vi "afonin_et7026(1) — 18.09.2023.vi"() -> ()   [LabVIEW 2012]
panel:
  out "error out":errorcluster
  out "Торр":dbl format="%#_2g"
  out "Па":dbl format="%#_2e"
  out "мбар":dbl format="%#_2g"
  out "Торр":dbl(graph)
  out "Waveform Chart":dbl(graph)
  in  "Remote Port":u16=502
  in  "Remote IP for 7026":string="127.0.0.1"
  in  "Stop":bool
  out "AI":u16[](array[numeric])
  out "DI":bool[](array[boolean]) caption="Slave Discrete Inputs"
  in  "DO":bool[](array[boolean])=[FALSE, FALSE, FALSE, FALSE] caption="Coils to Write"
  in  "AO":u16[](array[numeric])=[0, 0, 0, 0] caption="Registers to Write"
  # "192.168.0.122"
  # "Data to write to the slave"
  # "Slave Read-only Registers"
  # "DO 0"
  # "DO 1"
  # "DI 0"
  # "DI 1"
  # "AO 0"
  # "AO 1"
  # "AI 0"
  # "AI 1"
  # "AI 2"
  # "AI 3"
  # "AI 4"
  # "AI 5"
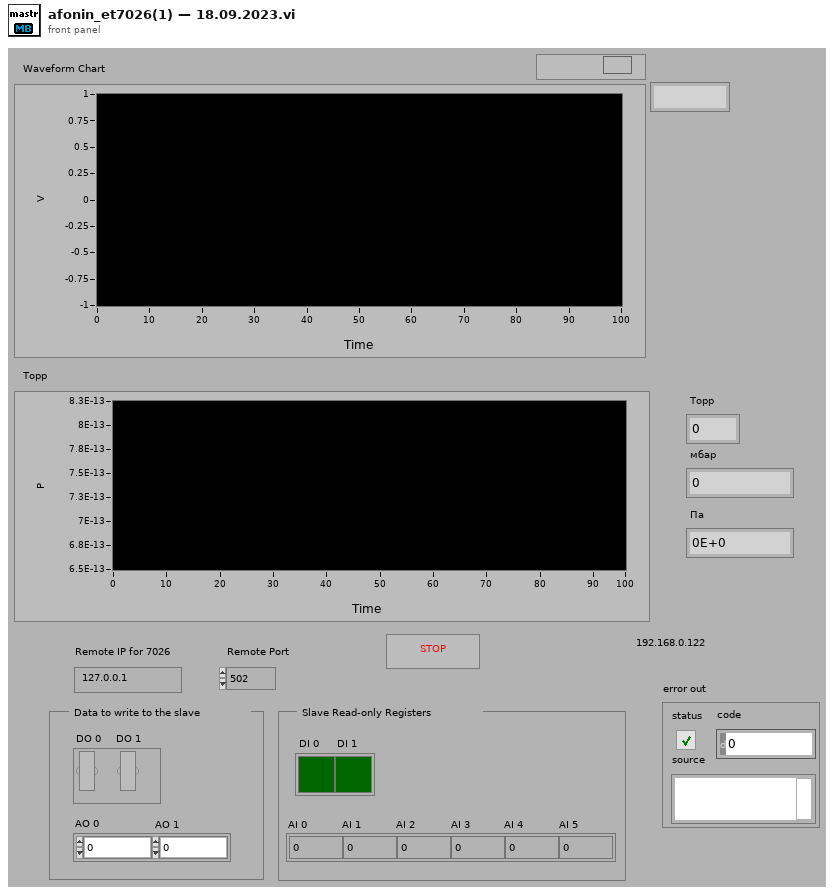
[diagram p1: front panel]
types:
  T1 = typedef "MB Modbus Command.ctl" = cluster{"Function Code":u8, "Starting Address":u16, "Quantity":u16, "Data":u16[], "Discrete":bool[]}
  T2 = enum16{"open", "replace", "create", "open or create", "replace or create", "replace or create with confirmation"}
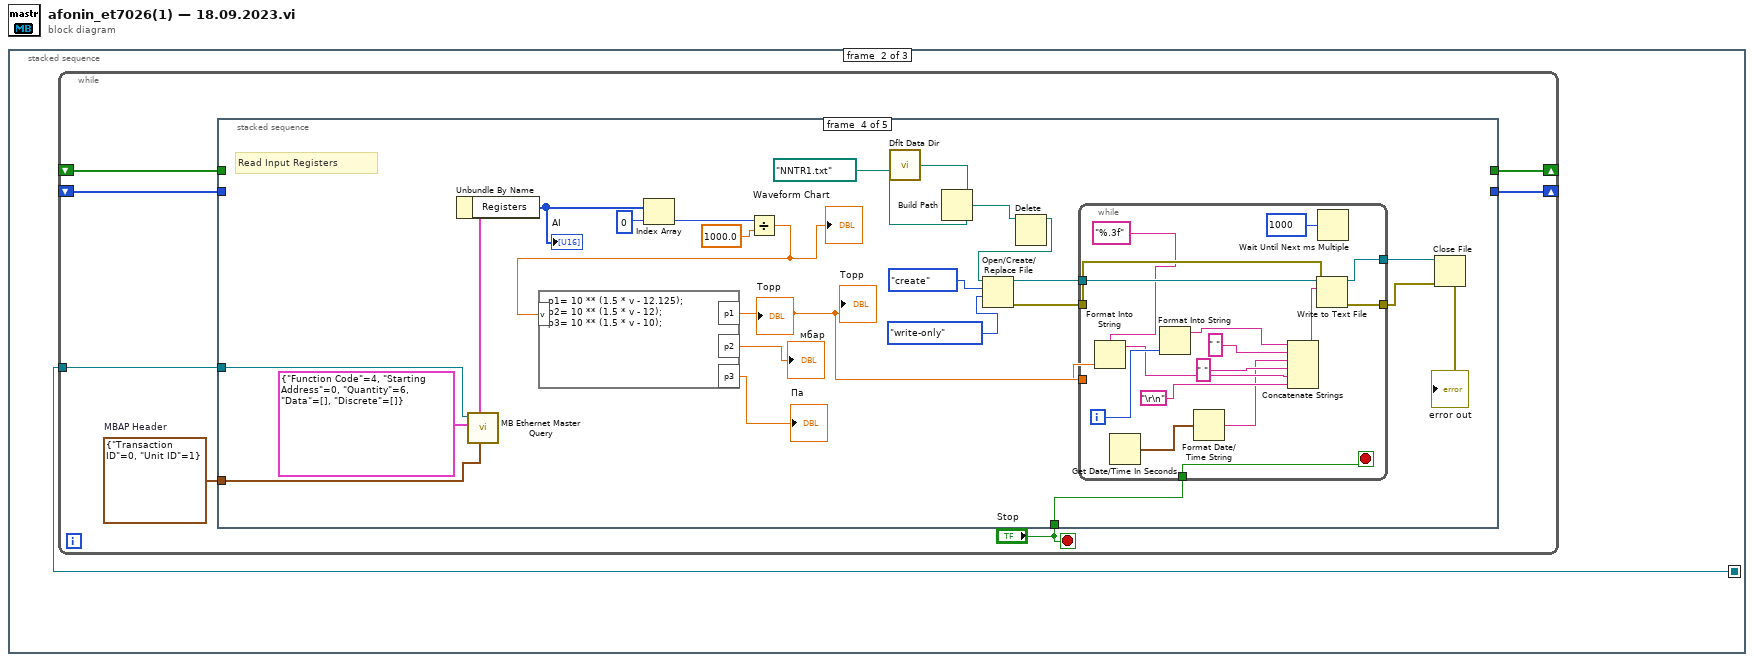
[diagram p0: block diagram]
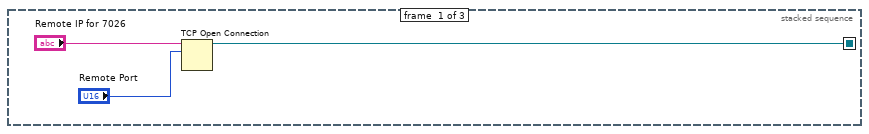
[diagram p2: hidden frame]
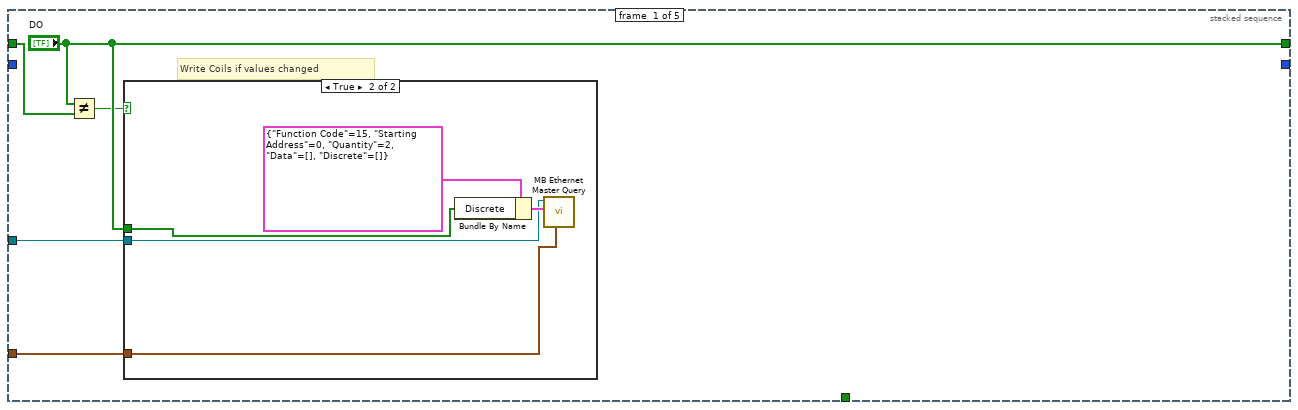
[diagram p3: hidden frame]
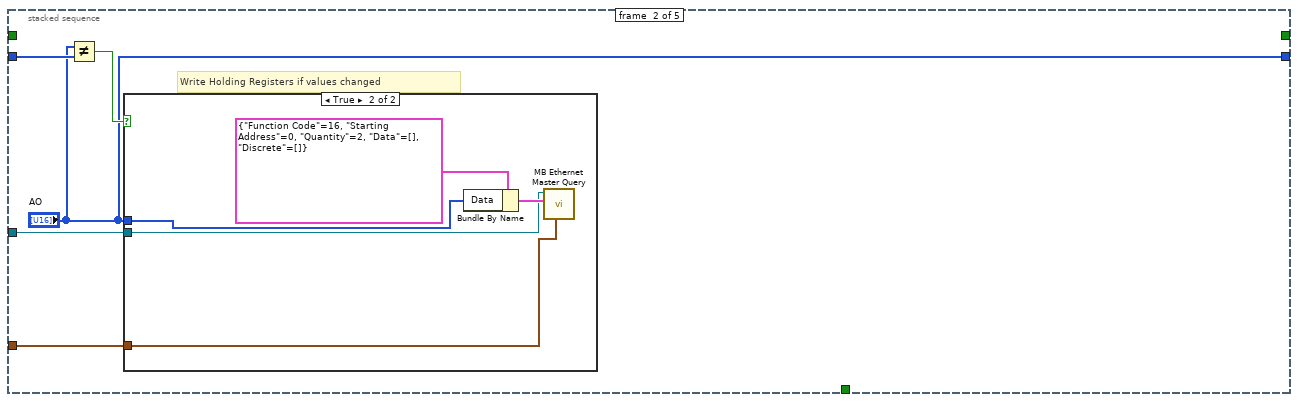
[diagram p5: hidden frame]
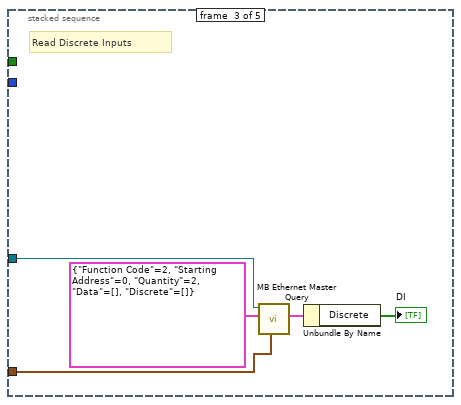
[diagram p7: hidden frame]
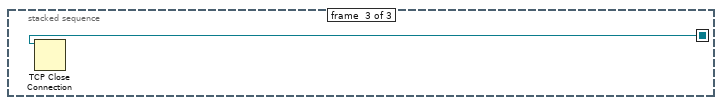
[diagram p9: hidden frame]
diagram:
  n1 = stacked-sequence {
    seq-local: [w1 _ _] -> [_ w4 w78]
    frame #0 {
      n2 = TCP Open Connection(address="Remote IP for 7026", remote port or service name="Remote Port") -> (connection ID=w1:refnum<k5>)  [unwired: 3 in, 1 out]
    }
    frame #1 {
      n3 = while {
        tunnel: w4 -> [w11]
        shift-right: [w9] -> _
        shift-left: _ -> [w10]
        shift-right: [w7] -> _
        shift-left: _ -> [w8]
        stop <- "Stop" stop-if-true
        w6 = cluster{"Transaction ID":u16, "Unit ID":u8} {"Transaction ID"=0, "Unit ID"=1}  # MBAP Header
        n4 = stacked-sequence {
          tunnel: w11 -> [w16 w26 w36 w60 _]
          tunnel: w10 -> [w15 _ _ _ _]
          tunnel: ["DO" _ _ _ _] -> w9
          tunnel: w8 -> [_ w24 _ _ _]
          tunnel: [_ "AO" _ _ _] -> w7
          tunnel: w6 -> [w12 w22 w32 w57 _]
          tunnel: "Stop" -> [_ _ _ w46 _]
          frame #0 {
            # "Write Coils if values changed"
            n5 = Not Equal?(x="DO", y=w15) -> (x != y?=w13:bool)
            n6 = case shown="True" w13 {
              tunnel: w16 -> [_ w19]
              tunnel: "DO" -> [_ w18]
              tunnel: w12 -> [_ w17]
              frame False {
              }
              frame True {
                n7 = Bundle By Name(cluster=T1 {"Function Code"=15, "Starting Address"=0, "Quantity"=2, "Data"=[], "Discrete"=[]} ("MODBUS Command"), "Discrete"=w18) -> (w20:T1)
                n8 = call "MB Ethernet Master Query.vi"("MBAP Header"=w17, "Modbus Command"=w20, "TCP Connection Refnum in"=w19) -> ()  [unwired: 4 in, 5 out]
              }
            }
          }
          frame #1 {
            # "Write Holding Registers if values changed"
            n9 = Not Equal?(x="AO", y=w24) -> (x != y?=w25:bool)
            n10 = case shown="True" w25 {
              tunnel: w26 -> [_ w29]
              tunnel: "AO" -> [_ w28]
              tunnel: w22 -> [_ w27]
              frame False {
              }
              frame True {
                n11 = Bundle By Name(cluster=T1 {"Function Code"=16, "Starting Address"=0, "Quantity"=2, "Data"=[], "Discrete"=[]} ("MODBUS Command"), "Data"=w28) -> (w30:T1)
                n12 = call "MB Ethernet Master Query.vi"("MBAP Header"=w27, "Modbus Command"=w30, "TCP Connection Refnum in"=w29) -> ()  [unwired: 4 in, 5 out]
              }
            }
          }
          frame #2 {
            # "Read Discrete Inputs"
            n13 = call "MB Ethernet Master Query.vi"("MBAP Header"=w32, "Modbus Command"=T1 {"Function Code"=2, "Starting Address"=0, "Quantity"=2, "Data"=[], "Discrete"=[]} ("MODBUS Command"), "TCP Connection Refnum in"=w36) -> ("Registers"=w35:cluster{"Registers":u16[], "Discrete":bool[]})  [unwired: 4 in, 4 out]
            n14 = Unbundle By Name(w35) -> ("Discrete"=→"DI":bool[])
          }
          frame #3 {
            # "Read Input Registers"
            n15 = call "MB Ethernet Master Query.vi"("MBAP Header"=w57, "Modbus Command"=T1 {"Function Code"=4, "Starting Address"=0, "Quantity"=6, "Data"=[], "Discrete"=[]} ("MODBUS Command"), "TCP Connection Refnum in"=w60) -> ("Registers"=w59:cluster{"Registers":u16[], "Discrete":bool[]})  [unwired: 4 in, 4 out]
            n16 = Unbundle By Name(w59) -> ("Registers"=w56:u16[])
            "AI" <- w56
            n17 = Index Array(array=w56, index=0) -> (element=w53:u16)
            n18 = Divide(x=w53, y=1000.0) -> (x/y=w52:dbl)
            "Waveform Chart" <- w52
            n19 = formula code="p1= 10 ** (1.5 * v - 12.125);\np2= 10 ** (1.5 * v - 12);\np3= 10 ** (1.5 * v - 10);"("v"=w52) -> ("p1"=w47:dbl, "p2"=→"мбар":dbl, "p3"=→"Па":dbl)
            "Торр" <- w47
            "Торр" <- w47
            n20 = call <vilib>:"Dflt Data Dir.vi"() -> ("App:Default Data Directory"=w45:path)
            n21 = Build Path(base path=w45, name or relative path=path "NNTR1.txt" ("Path")) -> (appended path=w44:path)
            n22 = Delete(path (use dialog)=w44) -> (deleted path=w43:path)  [unwired: 4 in, 2 out]
            n23 = Open/Create/Replace File(file path (use dialog)=w43, operation (0:open)=T2."create", access (0:read/write)=enum16{"read/write", "read-only", "write-only"}."write-only") -> (refnum out=w48:refnum<file>, error out=w42:errorcluster)  [unwired: 3 in, 1 out]
            n24 = while {
              tunnel: w48 -> [w77]
              tunnel: w47 -> [w76]
              tunnel: w46 -> [w73]
              tunnel: w42 -> [w71]
              tunnel: [w70] -> w41
              tunnel: [w69] -> w40
              i -> [w72]
              stop <- w73 stop-if-true
              n25 = Format Into String(format string="%.3f", w76) -> (resulting string=w62:string)  [unwired: 2 in, 1 out]
              n26 = Get Date/Time In Seconds() -> (seconds since 1Jan1904=w63:timestamp)
              n27 = Format Into String(w72) -> (resulting string=w66:string)  [unwired: 3 in, 1 out]
              n28 = Format Date/Time String(seconds (now)=w63) -> (date/time string=w61:string)  [unwired: 2 in]
              n29 = Concatenate Strings(w66, " " ("string"), w61, " " ("string"), w62, "\r\n") -> (w67:string)
              n30 = Write to Text File(file (use dialog)=w77, text=w67, error in=w71) -> (refnum out=w70:refnum<file>, error out=w69:errorcluster)  [unwired: 1 in, 1 out]
              n31 = Wait Until Next ms Multiple(millisecond multiple=u32 1000) -> ()  [unwired: 1 out]
            }
            n32 = Close File(refnum=w41, error in=w40) -> (error out=→"error out":errorcluster)  [unwired: 1 out]
          }
          frame #4 {
          }
        }
      }
    }
    frame #2 {
      n33 = TCP Close Connection(connection ID=w78) -> ()  [unwired: 2 in, 2 out]
    }
  }
